vi "All Headers.vi"(8 "error in (no error)":errorcluster, 11 "Response in":refnum<class "Response.lvclass">) -> (0 "error out":errorcluster, 2 "Headers":cluster{"Header":string, "Value":string}[](array[cluster]), 3 "Response out":refnum<class "Response.lvclass">)   [LabVIEW 2020, in "HTTP Utils.lvlib" / "Response.lvclass"]
uses:
  Response.lvclass
  Response.lvclass/Response.ctl
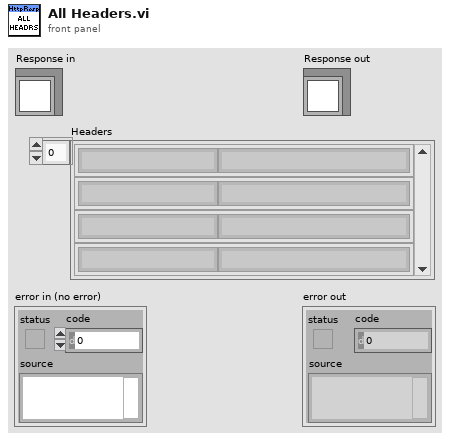
[diagram p1: front panel]
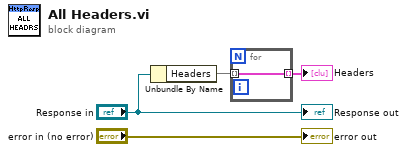
[diagram p0: block diagram]
diagram:
  n1 = Unbundle By Name("Response in") -> ("Headers"=w3:map{string, string})
  n2 = for {
    tunnel: w3 -> [w5] mode=indexing
    tunnel: [w5] -> w2 mode=indexing
  }
  "Headers" <- w2
  "error out" <- "error in (no error)"
  "Response out" <- "Response in"
